vi "Apply Memory Polynomial.vi"(0 "Instrument Handle In":refnum<k21>, 1 "Selector String":string, 5 "RFSG handle":refnum<k15>, 7 "Common Configuration":T3={"Measurement Interval (s)"=0.0001, "Sample Rate Mode"=1, "Sample Rate (Hz)"=120000000.0, "Signal Type"=0, "Pre DPD CFR Enabled"=0, "Apply DPD CFR Enabled"=0, "DUT Average Input Power (dBm)"=-15.0} {"DUT Average Input Power (dBm)" format="%.2f"; "Apply DPD CFR Enabled" items=["False", "True"]; "Pre DPD CFR Enabled" items=["False", "True"]; "Signal Type" items=["Modulated", "Tones"]; "Sample Rate (Hz)" format="%.2p"; "Sample Rate Mode" items=["User", "Reference Waveform"]; "Measurement Interval (s)" format="%#.2p"}, 9 "Waveform":T4={"Waveform Name"="Wfm", "Waveform"={"x0"=0.0, "dx"=0.0, "y"=[]}, "Signal Bandwidth (Hz)"=0.0, "PAPR (dB)"=0.0, "Burst Length (s)"=0.0, "Sample Rate"=0.0, "Burst Start Locations"=[], "Burst Stop Locations"=[], "Idle Duration Present?"=FALSE, "Runtime Scaling"=0.0} {"Runtime Scaling" format="%#_6p"; "Sample Rate" format="%#_6p"; "Burst Length (s)" format="%#_6p"; "PAPR (dB)" format="%.2f"; "Signal Bandwidth (Hz)" format="%#_6p"; "Waveform"."y" format="%.2f"; "Waveform"."dx" format="%^.2e"; "Waveform"."x0" format="%^.2e"}, 11 "error in (no error)":errorcluster, 12 "Memory Polynomial Configuration":T2={"Correction Type"=0, " Iterative DPD Enabled"=0, "Number of Iterations"=3, " Order"=3, " Depth"=2, "Maximum Lag"=2, "Maximum Lead"=2, "Lag Order"=2, "Lead Order"=2, "Lag Memory Depth"=2, "Lead Memory Depth"=2} {"Number of Iterations" min=1; "Iterative DPD Enabled" items=["False", "True"]; "Correction Type" items=["Magnitude and Phase", "Magnitude Only", "Phase Only"]}) -> (4 "Instrument Handle Out":refnum<k21>, 6 "RFSG instrument handle out":refnum<k15>, 8 "Memory Polynomial Results":T1={"Post Dpd Waveform"={"x0"=0.0, "dx"=0.0, "y"=[]}, "Post Dpd Papr (dB)"=-1.0, "Power Offset (dB)"=-1.0, "DPD Polynomial"=[]} {"DPD Polynomial" format="%.2f"; "Power Offset (dB)" format="%.2f"; "Post Dpd Papr (dB)" format="%.2f"; "Post Dpd Waveform"."y" format="%.2f"; "Post Dpd Waveform"."dx" format="%^.2e"; "Post Dpd Waveform"."x0" format="%^.2e"}, 15 "error out":errorcluster)   [LabVIEW 2016, in "RFmxDPD.lvlib"]
uses:
  RFmxDPD.lvlib
  SG/Typedefs/Waveform.ctl
  Typedefs/Common Configuration.ctl
  Typedefs/Memory Polynomial Configuration.ctl
  Typedefs/Memory Polynomial Results.ctl
  <vilib>/RFmx/SpecAn/mx/RFmxSpecAn.llb/RFmxSpecAn DPD Fetch DPD Polynomial.vi
  SG/SG.lvlib
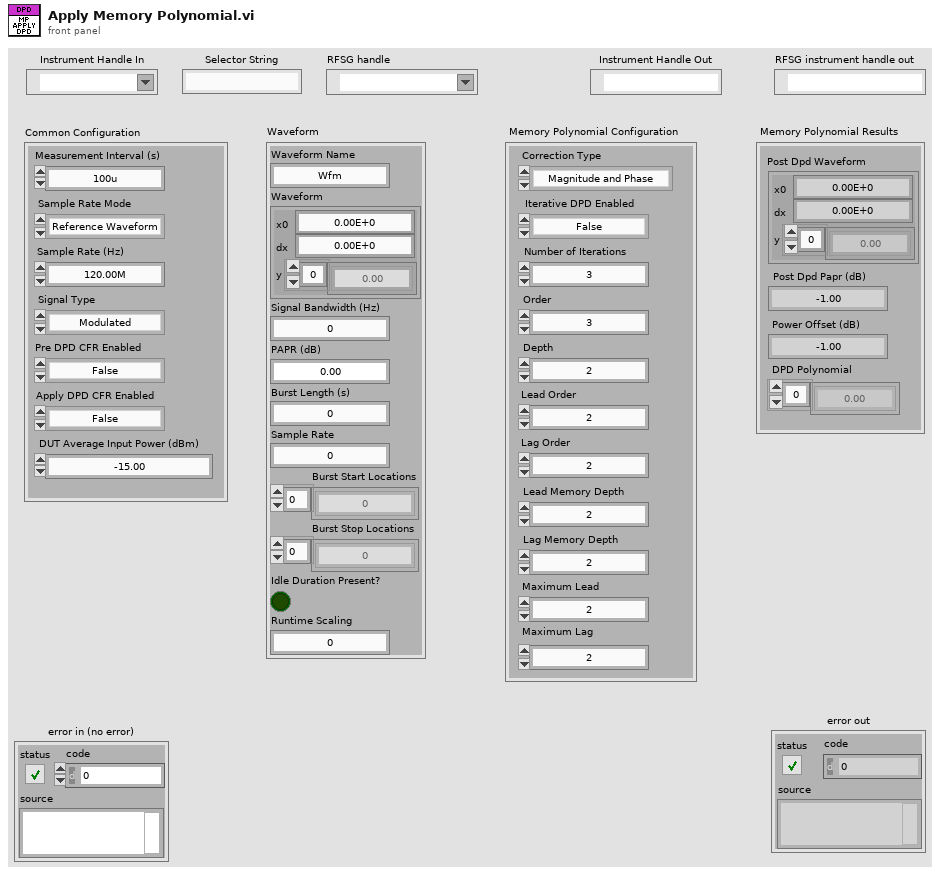
[diagram p1: front panel]
types:
  T1 = typedef "RFmxDPD.lvlib/Memory Polynomial Results.ctl" = cluster{"Post Dpd Waveform":cluster{"x0":dbl, "dx":dbl, "y":csg[]}, "Post Dpd Papr (dB)":dbl, "Power Offset (dB)":dbl, "DPD Polynomial":csg[]}
  T2 = typedef "RFmxDPD.lvlib/Memory Polynomial Configuration.ctl" = cluster{"Correction Type":i32, " Iterative DPD Enabled":i32, "Number of Iterations":i32, " Order":i32, " Depth":i32, "Maximum Lag":i32, "Maximum Lead":i32, "Lag Order":i32, "Lead Order":i32, "Lag Memory Depth":i32, "Lead Memory Depth":i32}
  T3 = typedef "RFmxDPD.lvlib/Common Configuration.ctl" = cluster{"Measurement Interval (s)":dbl, "Sample Rate Mode":i32, "Sample Rate (Hz)":dbl, "Signal Type":i32, "Pre DPD CFR Enabled":i32, "Apply DPD CFR Enabled":i32, "DUT Average Input Power (dBm)":dbl}
  T4 = typedef "SG.lvlib/Waveform.ctl" = cluster{"Waveform Name":string, "Waveform":cluster{"x0":dbl, "dx":dbl, "y":csg[]}, "Signal Bandwidth (Hz)":dbl, "PAPR (dB)":dbl, "Burst Length (s)":dbl, "Sample Rate":dbl, "Burst Start Locations":i32[], "Burst Stop Locations":i32[], "Idle Duration Present?":bool, "Runtime Scaling":dbl}
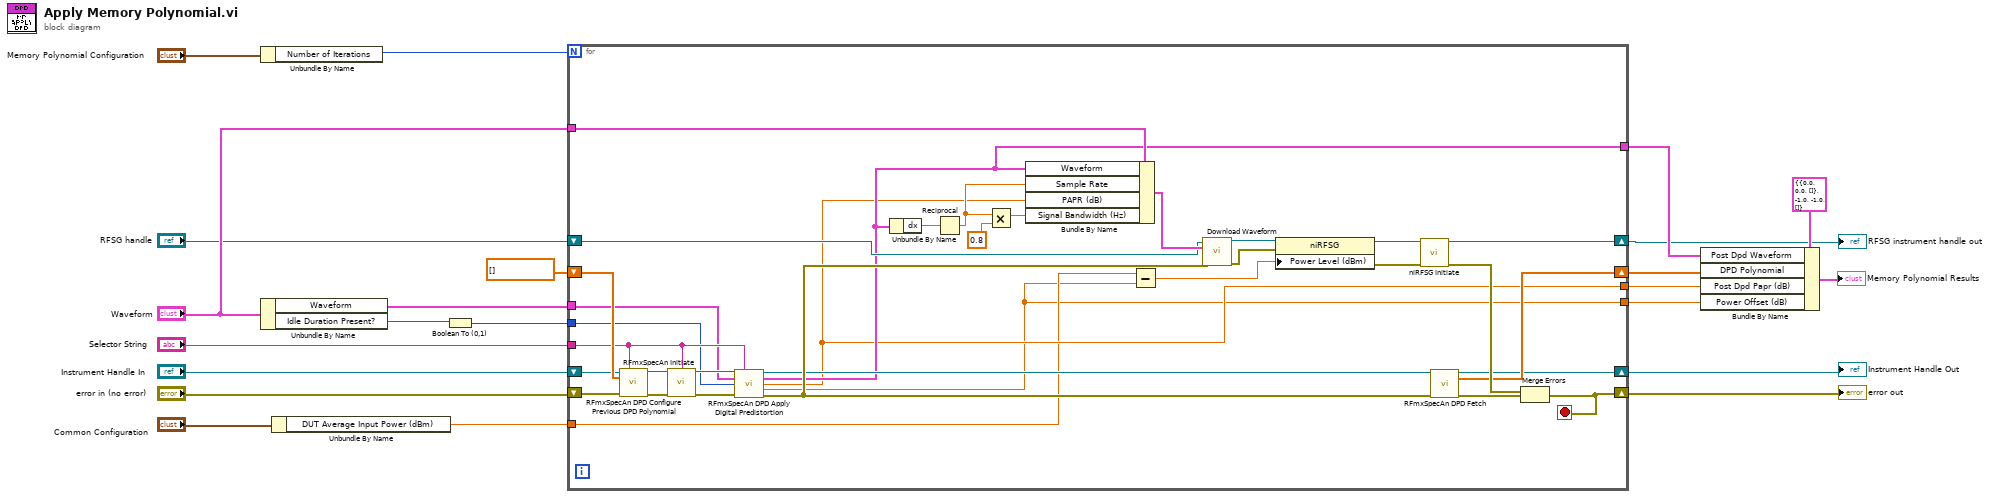
[diagram p0: block diagram]
diagram:
  n1 = Unbundle By Name("Memory Polynomial Configuration") -> ("Number of Iterations"=w12:i32)
  n2 = Unbundle By Name("Waveform") -> ("Waveform"=w16:cluster{"x0":dbl, "dx":dbl, "y":csg[]}, "Idle Duration Present?"=w18:bool)
  n3 = Unbundle By Name("Common Configuration") -> ("DUT Average Input Power (dBm)"=w15:dbl)
  n4 = Boolean To (0,1)(Boolean=w18) -> (0, 1=w17:i16)
  n5 = for {
    N: w12 -> [_]
    shift-right: [w26] -> w5
    shift-left: "Instrument Handle In" -> [w40]
    shift-right: [w56] -> w9
    shift-left: "error in (no error)" -> [w39]
    shift-right: [w29] -> w11
    shift-left: csg[] [] ("DPD Polynomial") -> [w54]
    tunnel: "Selector String" -> [w38]
    tunnel: w17 -> [w37]
    tunnel: w16 -> [w36]
    tunnel: w15 -> [w24]
    tunnel: "Waveform" -> [w33]
    shift-right: [w30] -> w4
    shift-left: "RFSG handle" -> [w31]
    tunnel: [w28] -> w10
    tunnel: [w23] -> w7
    tunnel: [w27] -> w6
    stop <- w56 stop-if-true
    n6 = call <vilib>:"RFmxSpecAn DPD Configure Previous DPD Polynomial.vi"("Instrument Handle In"=w40, "Selector String"=w38, "Previous DPD Polynomial"=w54, "error in (no error)"=w39) -> ("Instrument Handle Out"=w52:refnum<k21>, "error out"=w53:errorcluster)  [unwired: 10 in]
    n7 = call <vilib>:"RFmxSpecAn Initiate.vi"("Instrument Handle In"=w52, "Result Name"=w38, "error in (no error)"=w53) -> ("Instrument Handle Out"=w44:refnum<k21>, "error out"=w43:errorcluster)  [unwired: 10 in, 1 out]
    n8 = call <vilib>:"RFmxSpecAn DPD Apply Digital Predistortion.vi"("Instrument Handle In"=w44, "Selector String"=w38, "Waveform In"=w36, "Idle Duration Present"=w37, "error in (no error)"=w43) -> ("Instrument Handle Out"=w35:refnum<k21>, "Waveform Out"=w28:cluster{"x0":dbl, "dx":dbl, "y":csg[]}, "PAPR (dB)"=w27:dbl, "Power Offset (dB)"=w23:dbl, "error out"=w42:errorcluster)  [unwired: 6 in]
    n9 = Unbundle By Name(w28) -> ("dx"=w45:dbl)
    n10 = Reciprocal(x=w45) -> (1/x=w46:dbl)
    n11 = Multiply(x=w46, y=0.8) -> (x*y=w47:dbl)
    n12 = Bundle By Name(cluster=w33, "Waveform"=w28, "Sample Rate"=w46, "PAPR (dB)"=w27, "Signal Bandwidth (Hz)"=w47) -> (w32:T4)
    n13 = Subtract(x=w24, y=w23) -> (x-y=w25:dbl)
    n14 = call "Download Waveform.vi"("RFSG handle"=w31, "Waveform In"=w32, "error in (no error)"=w42) -> ("RFSG handle out"=w48:refnum<k15>, "error out"=w49:errorcluster)  [unwired: 11 in]
    n15 = property class="niRFSG"(reference=w48, error in=w49, "Power Level (dBm)"=w25) -> (reference out=w50:refnum<k15>, error out=w51:errorcluster)
    n16 = call <instrlib>:"niRFSG Initiate.vi"("instrument handle"=w50, "error in"=w51) -> ("instrument handle out"=w30:refnum<k15>, "error out"=w41:errorcluster)  [unwired: 12 in]
    n17 = call-poly <vilib>:"RFmxSpecAn DPD Fetch.vi"("Instrument Handle In"=w35, "error in (no error)"=w42) -> ("Instrument Handle Out"=w26:refnum<k21>, "DPD Polynomial"=w29:csg[], "error out"=w55:errorcluster)  [unwired: 11 in]
    n18 = Merge Errors(w41, w55) -> (w56:errorcluster)
  }
  "error out" <- w9
  "Instrument Handle Out" <- w5
  "RFSG instrument handle out" <- w4
  n19 = Bundle By Name(cluster=T1 {"Post Dpd Waveform"={"x0"=0.0, "dx"=0.0, "y"=[]}, "Post Dpd Papr (dB)"=-1.0, "Power Offset (dB)"=-1.0, "DPD Polynomial"=[]} ("RFmxMP Results"), "Post Dpd Waveform"=w10, "DPD Polynomial"=w11, "Post Dpd Papr (dB)"=w6, "Power Offset (dB)"=w7) -> (→"Memory Polynomial Results":T1)
